vi "Redis Server IP.vi"() -> (0 "server IP":string)   [LabVIEW 2019, in "Redis Client Examples.lvlib"]
uses:
  Redis Client Examples.lvlib
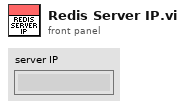
[diagram p1: front panel]
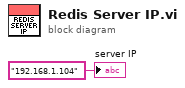
[diagram p0: block diagram]
diagram:
  "server IP" <- "192.168.1.104" ("server IP")
